vi "Linear Evaluation.vi"   [LabVIEW 2017, in "NI_AALPro.lvlib"]
doc: "Performs a linear evaluation on every element of <B>X</B> using the scale <B>a</B> and the offset <B>b</B>. Wire data to the <B>X</B> input to determine the polymorphic instance to use or manually select the instance."
uses:
  <vilib>/Analysis/NI_AALPro.lvlib
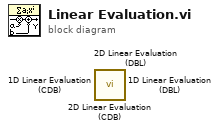
[diagram p0: block diagram]
diagram:
  n1 = call <vilib>:"2D Linear Evaluation (CDB).vi"() -> ()  [unwired: 3 in, 2 out]
  n2 = call <vilib>:"2D Linear Evaluation (DBL).vi"() -> ()  [unwired: 3 in, 2 out]
  n3 = call <vilib>:"1D Linear Evaluation (CDB).vi"() -> ()  [unwired: 3 in, 2 out]
  n4 = call <vilib>:"1D Linear Evaluation (DBL).vi"() -> ()  [unwired: 3 in, 2 out]
